vi "Autofocus Finish.vi"(8 "error in (no error)":errorcluster, 11 "Application in":refnum<class "Application.lvclass">) -> (0 "error out":errorcluster, 3 "Application out":refnum<class "Application.lvclass">)   [LabVIEW 2018, in "Application.lvlib" / "Application.lvclass"]
uses:
  Application.lvclass
  Application.lvclass/Application.ctl
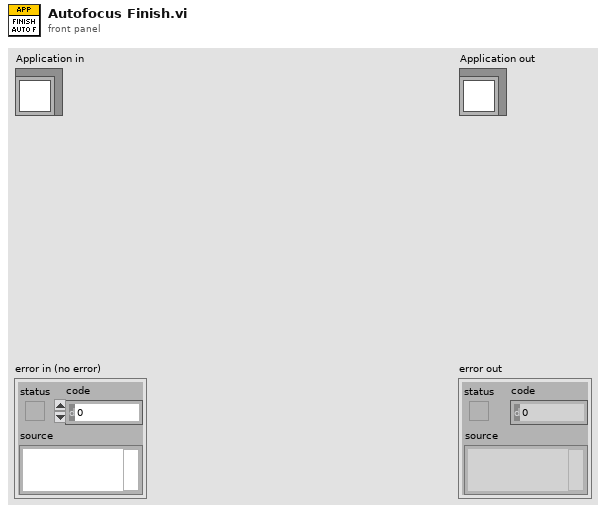
[diagram p1: front panel]
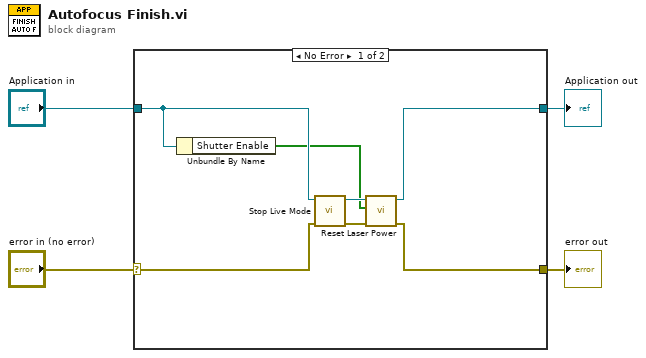
[diagram p0: block diagram]
diagram:
  n1 = case shown="No Error" "error in (no error)" {
    selector: "error in (no error)" -> [w11 w13]
    tunnel: [w8 w13] -> w3
    tunnel: [w9 w12] -> w1
    tunnel: "Application in" -> [w6 w12]
    frame No Error {
      n2 = Unbundle By Name(w6) -> ("Shutter Enable"=w5:bool[])
      n3 = call-dynamic "Stop Live Mode.vi"("error in (no error)"=w11, "Application in"=w6) -> ("error out"=w7:errorcluster, "Application out"=w10:refnum<class "Application.lvclass">)  [unwired: 8 in]
      n4 = call-dynamic "Reset Laser Power.vi"("error in (no error)"=w7, "Shutter Enable"=w5, "Application in"=w10) -> ("error out"=w8:errorcluster, "Application out"=w9:refnum<class "Application.lvclass">)  [unwired: 7 in]
    }
    frame Error {
    }
  }
  "error out" <- w3
  "Application out" <- w1
